vi "VWflipperArray.vi"(5 "Probe:Euler:Angles":T1, 6 "Probe Type":T2=5 items=["5-Hole Probe"=5, "OmniProbe"=12], 7 "Theta Degree":dbl[](array[numeric]), 8 "Probe w m/s":dbl[](array[numeric]), 9 "Probe v m/s":dbl[](array[numeric]), 10 "Probe u  m/s":dbl[](array[numeric]), 11 "VMagn m/s":dbl[](array[numeric])) -> (3 "VmagUVWCone":dbl[][](array[numeric]))   [LabVIEW 2021]
uses:
  Controls/AeroprobeType.ctl
  eulerAngles.ctl
  <vilib>/Analysis/coordinate.llb/Euler Rotation Order.ctl
  <vilib>/Analysis/coordinate.llb/3D Cartesian Coordinate Rotation (Euler) (Array).vi
  <vilib>/Analysis/NI_AALPro.lvlib
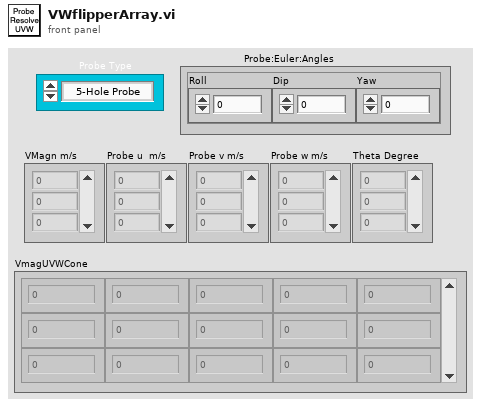
[diagram p1: front panel]
types:
  T1 = typedef "eulerAngles.ctl" = cluster{"Roll":dbl, "Dip":dbl, "Yaw":dbl}
  T2 = typedef "AeroprobeType.ctl" = u16
  T3 = typedef "NI_AALPro.lvlib/Euler Rotation Order.ctl" = u16
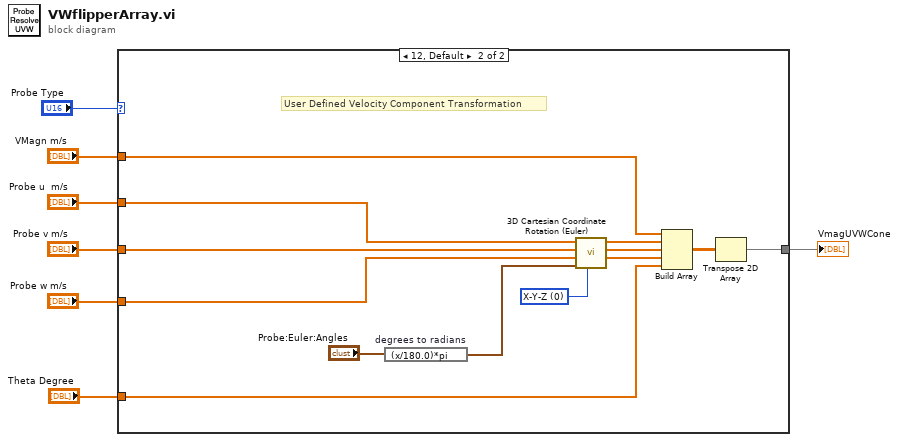
[diagram p0: block diagram]
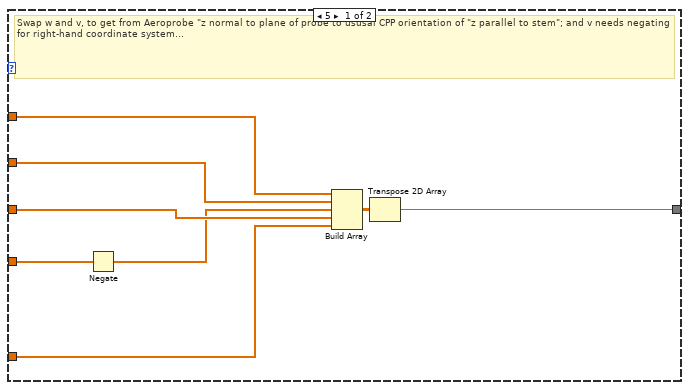
[diagram p2: hidden frame]
diagram:
  n1 = case shown="12, Default" "Probe Type" {
    tunnel: "Theta Degree" -> [w15 w28]
    tunnel: "Probe w m/s" -> [w14 w23]
    tunnel: "Probe v m/s" -> [w13 w24]
    tunnel: "Probe u  m/s" -> [w11 w27]
    tunnel: "VMagn m/s" -> [w10 w26]
    tunnel: [w8 w25] -> w2
    frame 5 {
      # "Swap w and v, to get from Aeroprobe \"z normal to plane of probe to ususal CPP orientation of \"z parallel to stem\"; and v needs negating for right-hand coordinate system..."
      n2 = Negate(x=w14) -> (-x=w12:dbl[])
      n3 = Build Array(w10, w11, w12, w13, w15) -> (w9:dbl[][])
      n4 = Transpose 2D Array(2D array=w9) -> (transposed array=w8:dbl[][])
    }
    frame 12, Default {
      w18 = T3 0 items=["X-Y-Z", "X-Z-Y", "Y-X-Z", "Y-Z-X", "Z-X-Y", "Z-Y-X", "X-Y-X", "X-Z-X", "Y-X-Y", "Y-Z-Y", "Z-X-Z", "Z-Y-Z"] ("rotation order")
      # "User Defined Velocity Component Transformation"
      n5 = expression code="(x/180.0)*pi" "degrees to radians"("Probe:Euler:Angles") -> (w16:T1)
      n6 = call-poly <vilib>:"3D Cartesian Coordinate Rotation (Euler).vi"("rotation order"=w18, "Euler Angles"=w16, "Z"=w23, "Y"=w24, "X"=w27) -> ("Z Out"=w19:dbl[], "Y Out"=w20:dbl[], "X Out"=w21:dbl[])  [unwired: 3 in, 1 out]
      n7 = Build Array(w26, w21, w20, w19, w28) -> (w22:dbl[][])
      n8 = Transpose 2D Array(2D array=w22) -> (transposed array=w25:dbl[][])
    }
  }
  "VmagUVWCone" <- w2
